vi "Write Bus type.vi"(8 "error in (no error)":errorcluster, 10 "Bus type":enum16{"Profibus DP", "Profibus PA"}(ring), 11 "Profibus in":refnum<class "Profibus.lvclass">) -> (0 "error out":errorcluster, 3 "Profibus out":refnum<class "Profibus.lvclass">)   [LabVIEW 2016, in "Profibus.lvclass"]
uses:
  Profibus.lvclass
  Profibus.lvclass/Profibus.ctl
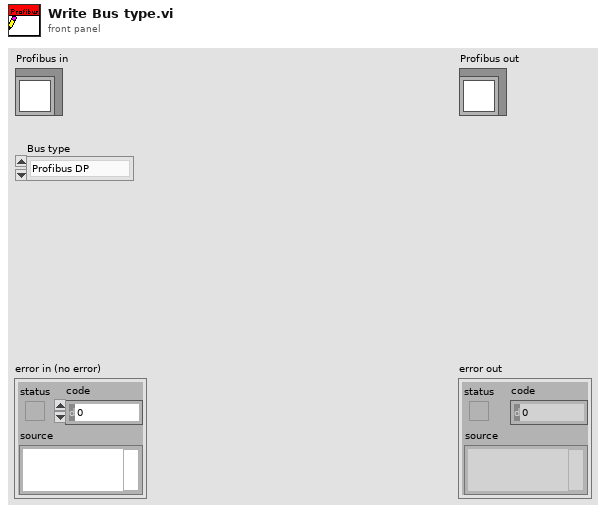
[diagram p1: front panel]
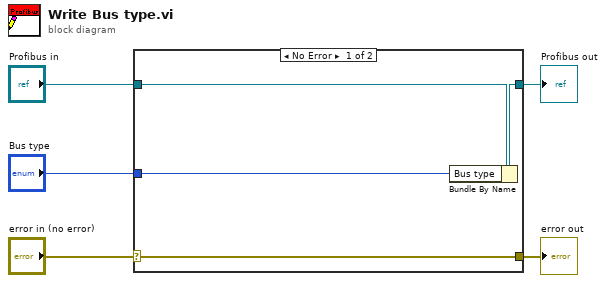
[diagram p0: block diagram]
diagram:
  n1 = case shown="No Error" "error in (no error)" {
    selector: "error in (no error)" -> [w9 w10]
    tunnel: [w9 w10] -> w4
    tunnel: [w7 w11] -> w2
    tunnel: "Profibus in" -> [w8 w11]
    tunnel: "Bus type" -> [w6 _]
    frame No Error {
      n2 = Bundle By Name(cluster=w8, "Bus type"=w6) -> (w7:refnum<class "Profibus.lvclass">)
    }
    frame Error {
    }
  }
  "error out" <- w4
  "Profibus out" <- w2
